vi "LVProjectShortcut_Item_OnDropItem.vi"(10 "DropItem":T1, 11 "Object":T1) -> ()   [LabVIEW 2017]
uses:
  <resource>/Framework/Providers/API/ItemRef.ctl
  <resource>/Framework/Providers/API/mxLvChangeType.ctl
  <resource>/Framework/Providers/API/mxLvUpdateUI.ctl
  <vilib>/Utility/lvfile.llb/NI_FileType.lvlib
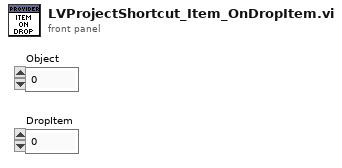
[diagram p1: front panel]
types:
  T1 = typedef "ItemRef.ctl" = u64
  T2 = typedef "mxLvUpdateUI.ctl" = cluster{"Action":u32, "Optional param 1":string, "Optional param 2":i32, "Optional param 3":string}
  T3 = typedef "mxLvChangeType.ctl" = enum32{"Item Created", "Item Modified", "File Modified", "File Deleted", "Item Added", "Item Added to SCC", "Item Renamed", "Item Modified For SCC"}
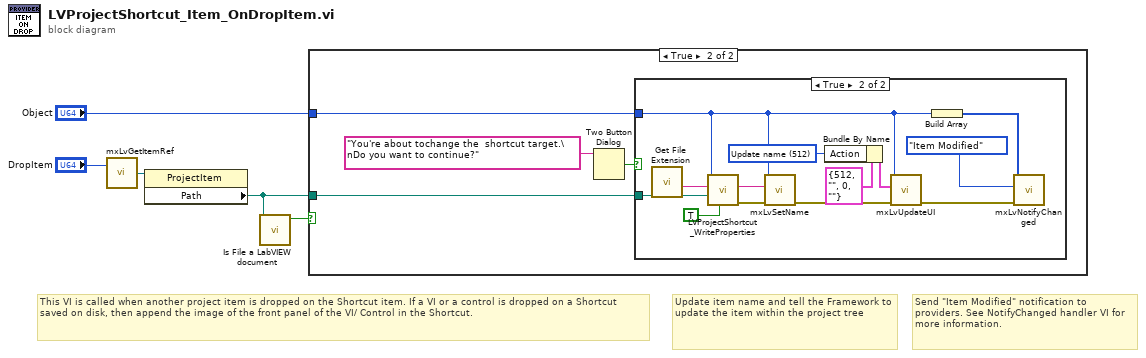
[diagram p0: block diagram]
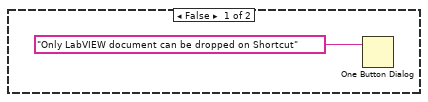
[diagram p2: hidden frame]
diagram:
  # "Update item name and tell the Framework to update the item within the project tree"
  # "Send \"Item Modified\" notification to providers. See NotifyChanged handler VI for more information."
  # "This VI is called when another project item is dropped on the Shortcut item. If a VI or a control is dropped on a Shortcut saved on disk, then append the image of the front panel of the VI/ Control in the Shortcut."
  n1 = call <resource>:"mxLvGetItemRef.vi"("Item"="DropItem") -> ("Item Refnum"=w4:refnum<vi>)  [unwired: 1 in, 2 out]
  n2 = property class="ProjectItem"(reference=w4) -> ("Path"=w2:path)  [unwired: 1 in, 2 out]
  n3 = call <vilib>:"Is File a LabVIEW document.vi"("path"=w2) -> ("Is LabVIEW document?"=w3:bool)  [unwired: 9 in, 1 out]
  n4 = case shown="True" w3 {
    tunnel: w2 -> [_ w9]
    tunnel: "Object" -> [_ w10]
    frame False {
      n5 = One Button Dialog(message="Only LabVIEW document can be dropped on Shortcut") -> ()  [unwired: 1 in, 1 out]
    }
    frame True {
      n6 = Two Button Dialog(message="You're about tochange the  shortcut target.\nDo you want to continue?") -> (T button?=w7:bool)  [unwired: 2 in]
      n7 = case shown="True" w7 {
        tunnel: w10 -> [_ w12]
        tunnel: w9 -> [_ w20]
        frame False {
        }
        frame True {
          w15 = u32 512 items=["Do nothing"=0, "Browse to item"=1, "Update item state"=2, "Update item icon"=4, "Activate view"=8, "Update view list"=16, "Expand item"=32, "Update child list"=64, "Update help"=128, "Refresh item 'F5'"=256, "Update name"=512, "Update menus and toolbars"=1024, "Update all user interface"=1494] ("Action")
          n8 = call <vilib>:"Get File Extension.vi"("file"=w20) -> ("filename without extension"=w11:string)  [unwired: 6 in, 4 out]
          n9 = call "LVProjectShortcut_WriteProperties.vi"("hasPath"=TRUE, "filePath"=w20, "shortcutName"=w11, "Wizard"=w12) -> ("error out"=w14:errorcluster)  [unwired: 7 in]
          n10 = call <resource>:"mxLvSetName.vi"("error in"=w14, "Name"=w11, "Item"=w12) -> ("error out"=w13:errorcluster)  [unwired: 7 in, 1 out]
          n11 = Bundle By Name(cluster=T2 {"Action"=512, "Optional param 1"="", "Optional param 2"=0, "Optional param 3"=""} ("Update UI Settings"), "Action"=w15) -> (w16:T2)
          n12 = call <resource>:"mxLvUpdateUI.vi"("error in"=w13, "Update UI Settings"=w16, "Item"=w12) -> ("error out"=w18:errorcluster)  [unwired: 7 in, 1 out]
          n13 = Build Array(w12) -> (w22:T1[])
          n14 = call <resource>:"mxLvNotifyChanged.vi"("error in (no error)"=w18, "Change Type"=mxLvChangeType."Item Modified", "Items"=w22) -> ()  [unwired: 7 in, 2 out]
        }
      }
    }
  }
